vi "testEXT Failes If Array Is Empty.vi"(8 "error in (no error)":errorcluster, 11 "TestCase in":refnum<class "Search In 1D Array Test Case.lvclass">) -> (0 "error out":errorcluster, 3 "TestCase out":refnum<class "Search In 1D Array Test Case.lvclass">)   [LabVIEW 2015, in "Search In 1D Array Test Case.lvclass"]
uses:
  Search In 1D Array Test Case.lvclass
  SubVIs/Search in array/Pass If In 1D Array (EXT).vi
  <vilib>/addons/_JKI Toolkits/VI Tester/TestCase.llb/TestCase.lvclass
  VITAC.lvlib
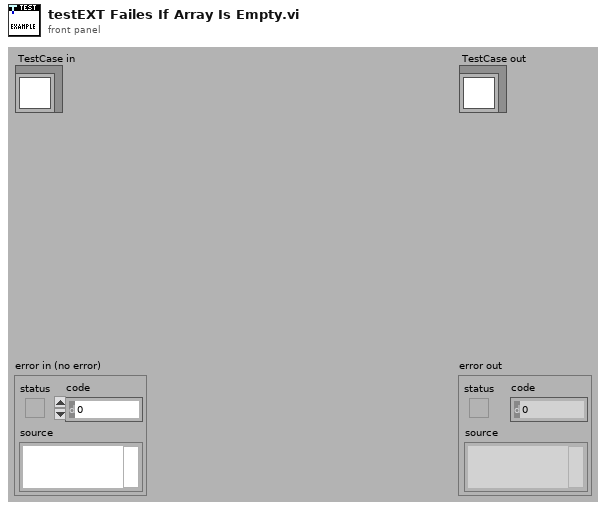
[diagram p1: front panel]
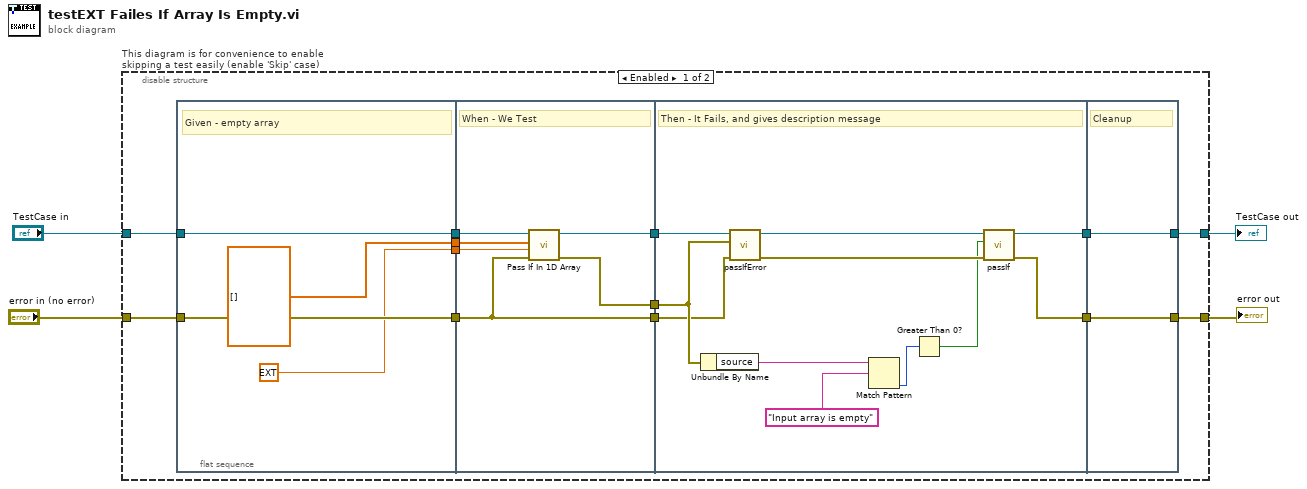
[diagram p0: block diagram]
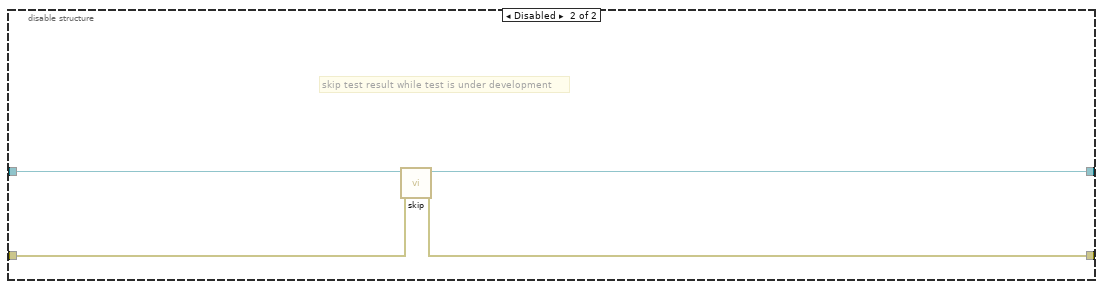
[diagram p2: hidden frame]
diagram:
  n1 = disable-structure "This diagram is for convenience to enable skipping a test easily (enable 'Skip' case)" shown="Enabled" {
    disable-tunnel: "TestCase in" -> [w9 w44]
    disable-tunnel: [w12 w42] -> w1
    disable-tunnel: [w11 w43] -> w3
    disable-tunnel: "error in (no error)" -> [w10 w41]
    frame Enabled {
      n2 = flat-sequence {
        tunnel: w10 -> [w20]
        tunnel: w9 -> [w21]
        tunnel: [w21] -> w17
        tunnel: [w20] -> w16
        tunnel: [ext 5.0] -> w8
        tunnel: [ext[] []] -> w7
        tunnel: [w26] -> w15
        tunnel: [w25] -> w14
        tunnel: w17 -> [w27]
        tunnel: w16 -> [w22]
        tunnel: w8 -> [w24]
        tunnel: w7 -> [w23]
        tunnel: [w22] -> w6
        tunnel: [w29] -> w13
        tunnel: w15 -> [w32]
        tunnel: w14 -> [w31]
        tunnel: w6 -> [w30]
        tunnel: [w28] -> w5
        tunnel: [w39] -> w11
        tunnel: [w40] -> w12
        tunnel: w13 -> [w40]
        tunnel: w5 -> [w39]
        frame #0 {
          # "Given - empty array"
        }
        frame #1 {
          # "When - We Test"
          n3 = call-poly "Pass If In 1D Array.vi"("error in (no error)"=w22, "element"=w24, "1D array"=w23, "TestCase in"=w27) -> ("error out"=w25:errorcluster, "TestCase out"=w26:refnum<class "Search In 1D Array Test Case.lvclass">)  [unwired: 6 in]
        }
        frame #2 {
          # "Then - It Fails, and gives description message"
          n4 = Unbundle By Name(w31) -> ("source"=w36:string)
          n5 = call-dynamic "passIfError.vi"("error in (no error)"=w30, "error"=w31, "TestCase in"=w32) -> ("error out"=w37:errorcluster, "TestCase out"=w38:refnum<class "Search In 1D Array Test Case.lvclass">)  [unwired: 7 in]
          n6 = Match Pattern(string=w36, regular expression="Input array is empty") -> (offset past match=w34:i32)  [unwired: 1 in, 3 out]
          n7 = Greater Than 0?(x=w34) -> (x > 0?=w33:bool)
          n8 = call-dynamic "passIf.vi"("error in (no error)"=w37, "pass"=w33, "TestCase in"=w38) -> ("error out"=w28:errorcluster, "TestCase out"=w29:refnum<class "Search In 1D Array Test Case.lvclass">)  [unwired: 7 in]
        }
        frame #3 {
          # "Cleanup"
        }
      }
    }
    frame Disabled {
      # "skip test result while test is under development"
      n9 = call <vilib>:"skip.vi"("error in (no error)"=w41, "TestCase in"=w44) -> ("error out"=w43:errorcluster, "TestCase out"=w42:refnum<class "Search In 1D Array Test Case.lvclass">)  [unwired: 8 in]
    }
  }
  "error out" <- w3
  "TestCase out" <- w1
